vi "ControlVoltage.vi"() -> ()   [LabVIEW 2017]
uses:
  <vilib>/Analysis/baseanly.llb/Mean (DBL).vi
  PowerMeter_Measurement.vi
  VoltageQueue_Global.vi
  MessageQueue/QueueOperations/Enqueue Message (Single).vi
  MessageQueue/MessageQueue.lvlib
  <vilib>/Analysis/NI_AALBase.lvlib
panel:
  in  "Initial Voltage":dbl
  out "mean":dbl format="%0.2f"
  out "standard deviation":dbl format="%0.2f"
  in  "Power (mW)":dbl
  in  "T (ms)":i32
  out "XY Graph":cluster{dbl[], dbl[]}(graph)
  in  "dt (ms)":u32=10
  in  "length":i32=10000
  in  "stop":bool
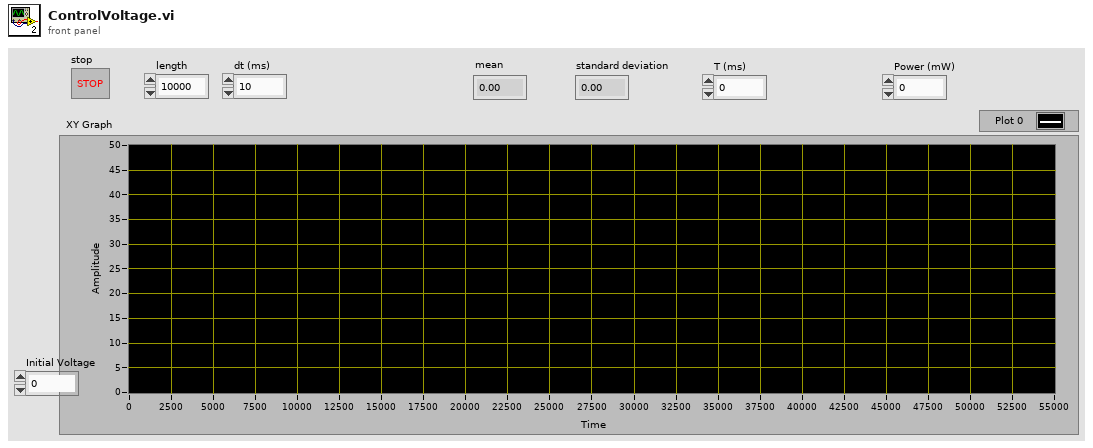
[diagram p1: front panel]
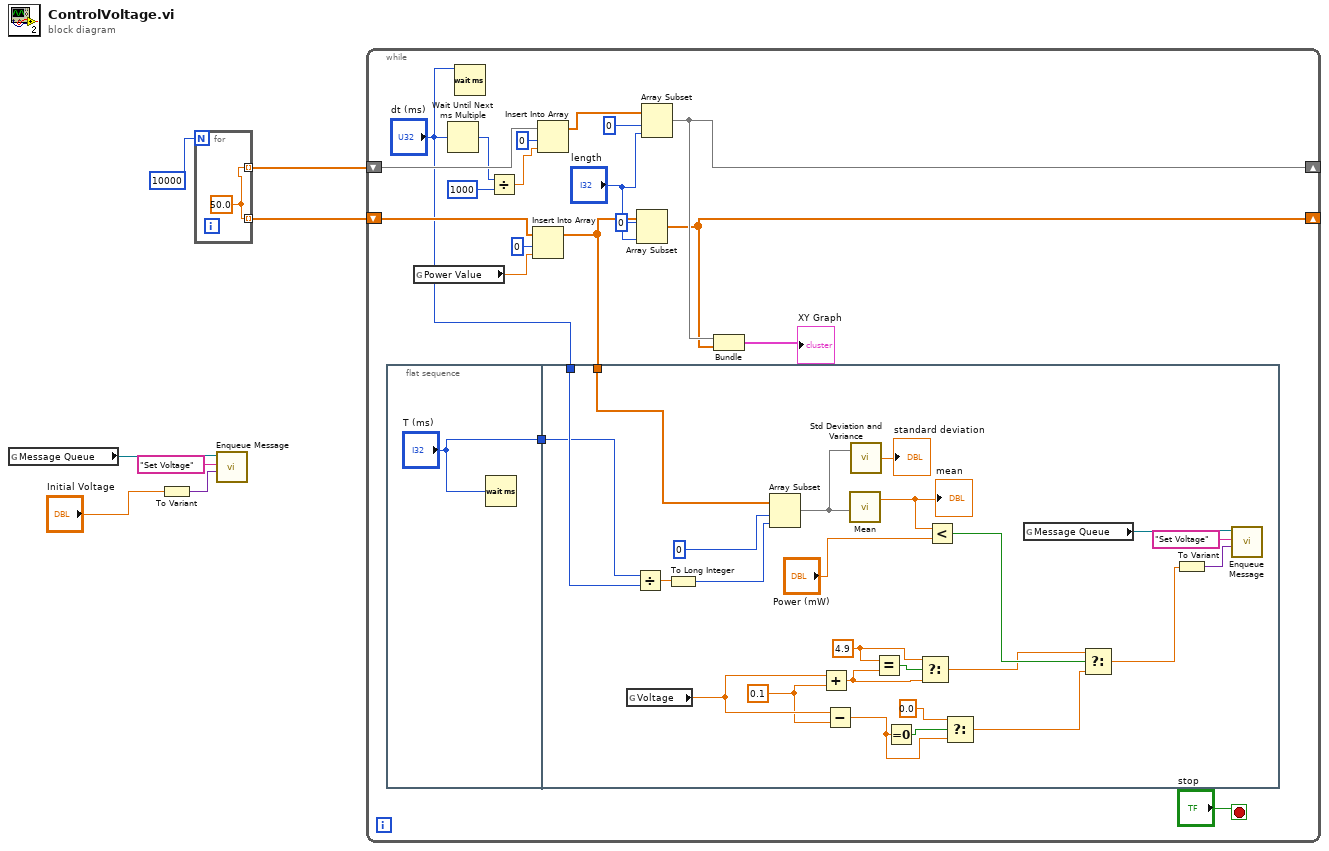
[diagram p0: block diagram]
diagram:
  n1 = global read "VoltageQueue_Global.vi" "Message Queue"() -> (w4:refnum<queue>)
  n2 = To Variant(anything="Initial Voltage") -> (Variant=w3:variant)
  n3 = for {
    N: 10000 -> [_]
    tunnel: [w8] -> w5 mode=indexing
    tunnel: [w8] -> w6 mode=indexing
    w8 = 50.0
  }
  n4 = call-poly "Enqueue Message.vi"("Message Data"=w3, "Message"="Set Voltage", "Message Queue"=w4) -> ()  [unwired: 7 in, 2 out]
  n5 = while {
    shift-right: [w15] -> _
    shift-left: w5 -> [w12]
    shift-right: [w21] -> _
    shift-left: w6 -> [w22]
    stop <- "stop" stop-if-true
    n6 = flat-sequence {
      tunnel: ["T (ms)"] -> w10
      tunnel: "dt (ms)" -> [w40]
      tunnel: w11 -> [w39]
      tunnel: w10 -> [w38]
      frame #0 {
        n7 = Wait (ms)(milliseconds to wait="T (ms)") -> ()  [unwired: 1 out]
      }
      frame #1 {
        w31 = 4.9 ("y")
        w42 = 0.1 ("y")
        n8 = global read "VoltageQueue_Global.vi" "Voltage"() -> (w43:dbl)
        n9 = Divide(x=w38, y=w40) -> (x/y=w51:dbl)
        n10 = To Long Integer(number=w51) -> (32bit integer=w50:i32)
        n11 = Array Subset(array=w39, index=0, length=w50) -> (w47:dbl[])
        n12 = Add(x=w43, y=w42) -> (x+y=w30:dbl)
        n13 = Subtract(x=w43, y=w42) -> (x-y=w36:dbl)
        n14 = call-poly <vilib>:"Mean.vi"("X"=w47) -> ("mean"=w49:dbl)  [unwired: 1 out]
        "mean" <- w49
        n15 = call <vilib>:"Std Deviation and Variance.vi"("X"=w47) -> ("standard deviation"=→"standard deviation":dbl)  [unwired: 1 in, 2 out]
        n16 = Equal?(x=w31, y=w30) -> (x = y?=w33:bool)
        n17 = Equal To 0?(x=w36) -> (x = 0?=w37:bool)
        n18 = Select(t=w31, s=w33, f=w30) -> (s? t:f=w32:dbl)
        n19 = Less?(x=w49, y="Power (mW)") -> (x < y?=w52:bool)
        n20 = Select(t=0.0 ("y"), s=w37, f=w36) -> (s? t:f=w34:dbl)
        n21 = global read "VoltageQueue_Global.vi" "Message Queue"() -> (w46:refnum<queue>)
        n22 = Select(t=w32, s=w52, f=w34) -> (s? t:f=w41:dbl)
        n23 = To Variant(anything=w41) -> (Variant=w45:variant)
        n24 = call-poly "Enqueue Message.vi"("Message Data"=w45, "Message"="Set Voltage", "Message Queue"=w46) -> ()  [unwired: 7 in, 2 out]
      }
    }
    n25 = global read "PowerMeter_Measurement.vi" "Power Value"() -> (w14:dbl)
    n26 = Wait Until Next ms Multiple(millisecond multiple="dt (ms)") -> (millisecond timer value=w17:u32)
    n27 = Wait (ms)(milliseconds to wait="dt (ms)") -> ()  [unwired: 1 out]
    n28 = Divide(x=w17, y=u32 1000) -> (x/y=w16:dbl)
    n29 = Insert Into Array(array=w12, index=0, new element=w14) -> (w11:dbl[])
    n30 = Insert Into Array(array=w22, index=0, new element=w16) -> (w25:dbl[])
    n31 = Array Subset(array=w11, index=0, length="length") -> (w15:dbl[])
    n32 = Array Subset(array=w25, index=0, length="length") -> (w21:dbl[])
    n33 = Bundle(w21, w15) -> (→"XY Graph":cluster{dbl[], dbl[]})  [unwired: 1 in]
  }
